vi "ReadPowerEnergyFile.vi"(1 "本次文件名":string) -> ()   [LabVIEW 2018]
uses:
  Init/AllPath.vi
  <vilib>/Utility/file.llb/Read Delimited Spreadsheet (string).vi
  HistoryFile.vi
panel:
  out "功率":string
  out "能量":string
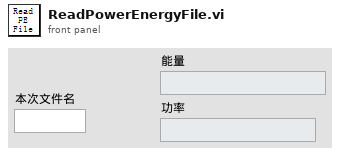
[diagram p1: front panel]
types:
  T1 = cluster{"能量/功率":path, " 示波器":path, " 光谱仪":path, "偏振":path, "近远场":cluster{" 近场图片":path, " 远场图片":path, "发散角数据":path}, "参数":path, " 基路径":path, "文件名信息":path}
  T2 = cluster{"能量计结果":string, "功率计结果":string, "能量计单位":string, " 功率计单位":string}
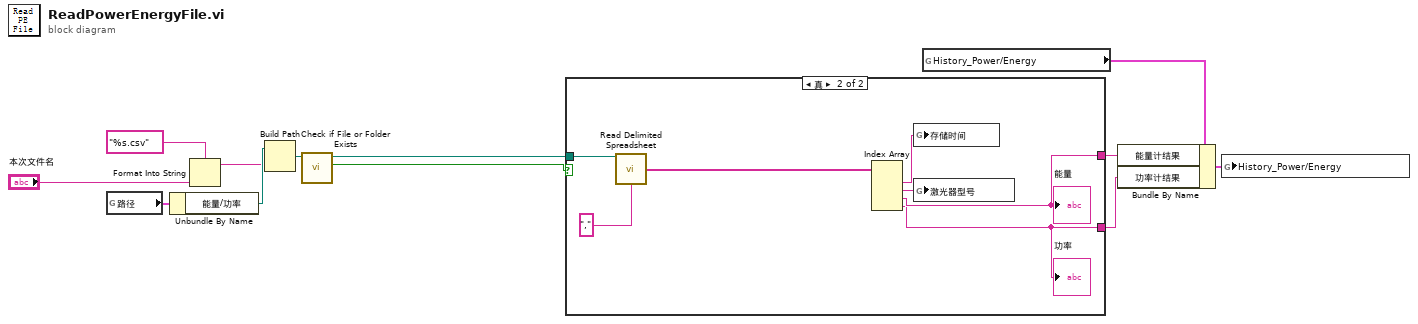
[diagram p0: block diagram]
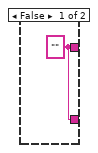
[diagram p2: hidden frame]
diagram:
  n1 = global read "AllPath.vi" "路径"() -> (w12:T1)
  n2 = Unbundle By Name(w12) -> ("能量/功率"=w11:path)
  n3 = Format Into String(format string="%s.csv" ("格式字符串"), "本次文件名") -> (resulting string=w8:string)  [unwired: 2 in, 1 out]
  n4 = Build Path(base path=w11, name or relative path=w8) -> (appended path=w3:path)
  n5 = call <vilib>:"Check if File or Folder Exists.vi"("path"=w3) -> ("file or folder exists?"=w1:bool, "dup path"=w2:path)  [unwired: 8 in, 1 out]
  n6 = case shown="真" w1 {
    tunnel: w2 -> [_ w20]
    tunnel: [w13 w17] -> w5
    tunnel: [w13 w16] -> w4
    frame False {
      w13 = ""
    }
    frame True {
      n7 = call-poly <vilib>:"Read Delimited Spreadsheet.vi"("file path (dialog if empty)"=w20, "delimiter (\\t)"="," ("delimiter (\\t)")) -> ("first row"=w19:string[])  [unwired: 8 in, 5 out]
      n8 = Index Array(array=w19) -> (element #1=w15:string, element #2=w14:string, element #3=w17:string, element #4=w16:string)  [unwired: 4 in]
      "能量" <- w17
      "功率" <- w16
      n9 = global write "HistoryFile.vi" "存储时间"(w15) -> ()
      n10 = global write "HistoryFile.vi" "激光器型号"(w14) -> ()
    }
  }
  n11 = global read "HistoryFile.vi" "History_Power/Energy"() -> (w7:T2)
  n12 = Bundle By Name(cluster=w7, "能量计结果"=w5, "功率计结果"=w4) -> (w6:T2)
  n13 = global write "HistoryFile.vi" "History_Power/Energy"(w6) -> ()
